vi "Check Status.vi"(8 "error in (no error)":errorcluster, 11 "Status Code":i32) -> (0 "error out":errorcluster, 3 "Error?":bool)   [LabVIEW 2018, in "PicoScope 3000a.lvlib" / "PicoScope 3000a.lvclass"]
uses:
  PicoScope 3000a.lvclass
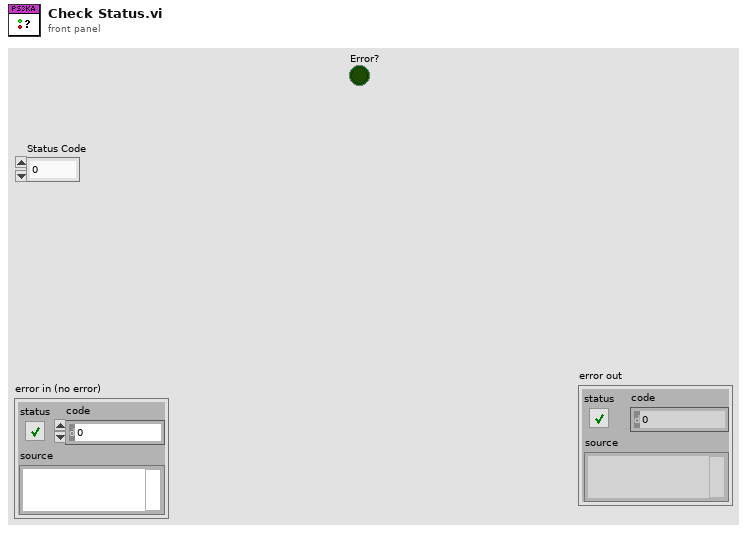
[diagram p1: front panel]
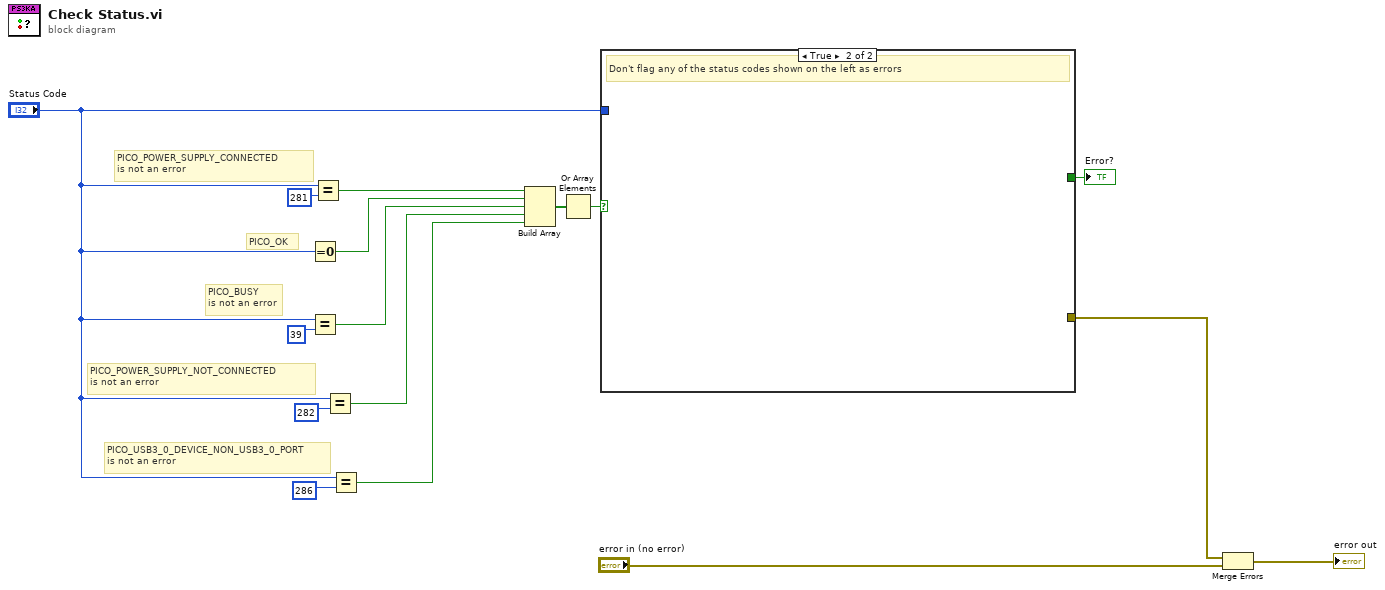
[diagram p0: block diagram]
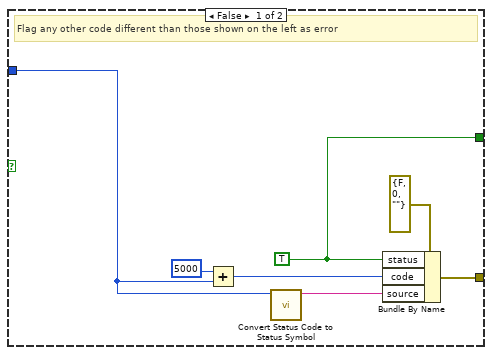
[diagram p2: hidden frame]
diagram:
  # "PICO_OK"
  # "PICO_USB3_0_DEVICE_NON_USB3_0_PORT\nis not an error"
  # "PICO_POWER_SUPPLY_CONNECTED \nis not an error"
  # "PICO_POWER_SUPPLY_NOT_CONNECTED \nis not an error"
  # "PICO_BUSY \nis not an error"
  n1 = Equal To 0?(x="Status Code") -> (x = 0?=w8:bool)
  n2 = Equal?(x="Status Code", y=39) -> (x = y?=w7:bool)
  n3 = Equal?(x="Status Code", y=281) -> (x = y?=w13:bool)
  n4 = Equal?(x="Status Code", y=282) -> (x = y?=w12:bool)
  n5 = Equal?(x="Status Code", y=286) -> (x = y?=w9:bool)
  n6 = Build Array(w13, w8, w7, w12, w9) -> (w11:bool[])
  n7 = Or Array Elements(Boolean array=w11) -> (logical OR=w6:bool)
  n8 = case shown="True" w6 {
    tunnel: "Status Code" -> [w19 _]
    tunnel: [w20 _] -> w2
    tunnel: [w17 _] -> w1
    frame False {
      w17 = TRUE ("status")
      # "Flag any other code different than those shown on the left as error"
      n9 = Add(x=5000, y=w19) -> (x+y=w22:i32)
      n10 = call "Convert Status Code to Status Symbol.vi"("Status Code"=w19) -> ("Status String"=w18:string)  [unwired: 9 in, 1 out]
      n11 = Bundle By Name(cluster=errorcluster {"status"=FALSE, "code"=0, "source"=""} ("error constant"), "status"=w17, "code"=w22, "source"=w18) -> (w20:errorcluster)
    }
    frame True {
      # "Don't flag any of the status codes shown on the left as errors"
    }
  }
  "Error?" <- w1
  n12 = Merge Errors(w2, "error in (no error)") -> (→"error out":errorcluster)
